vi "Harmonics MSMT Configure 5668 SA Pin.vi"(8 "error in (no error)":errorcluster, 11 "Harmonics in":refnum<class "Harmonics.lvclass">) -> (0 "error out":errorcluster, 2 "Original SA Pin":string, 3 "Harmonics out":refnum<class "Harmonics.lvclass">)   [LabVIEW 2018, in "Harmonics.lvlib" / "Harmonics.lvclass"]
uses:
  Harmonics.lvclass
  C:/Sequence Automation/Plugins/Measurement Interface.lvlibp/Measurement Interface.lvclass
  Plugins/Measurement Interface.lvlibp/Private Methods/Measurement Parameters/Read Measurement Parameters.vi
  Plugins/Measurement Interface.lvlibp/Private Methods/Measurement Parameters/Write Measurement Parameters.vi
  Plugins/String Database.lvlibp/String Database.lvclass
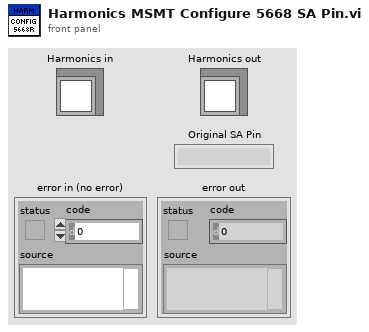
[diagram p1: front panel]
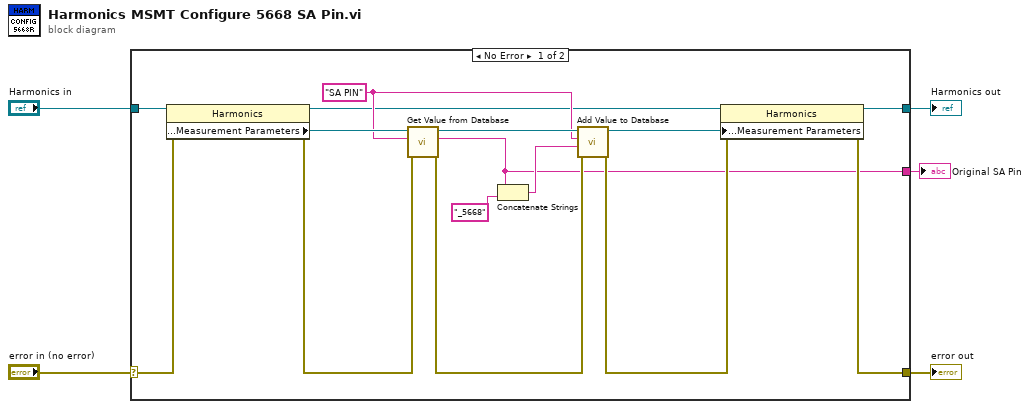
[diagram p0: block diagram]
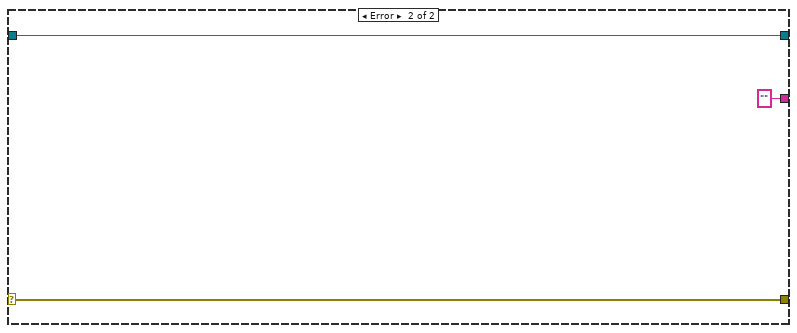
[diagram p2: hidden frame]
diagram:
  n1 = case shown="No Error" "error in (no error)" {
    selector: "error in (no error)" -> [w20 w23]
    tunnel: [w10 w23] -> w4
    tunnel: [w8 w22] -> w2
    tunnel: "Harmonics in" -> [w19 w22]
    tunnel: [w6 "" ("Entry Value")] -> w1
    frame No Error {
      w13 = "SA PIN" ("Entry Name")
      n2 = property class="Harmonics"(reference=w19, error in=w20) -> (reference out=w9:refnum<class "Harmonics.lvclass">, error out=w17:errorcluster, "Protected Methods:Measurement Parameters"=w18:refnum<class "String Database.lvclass">)
      n3 = call "Get Value from Database.vi"("error in (no error)"=w17, "Entry Name"=w13, "Message in"=w18) -> ("error out"=w12:errorcluster, "Entry Value"=w6:string, "Message out"=w15:refnum<class "String Database.lvclass">)  [unwired: 5 in, 1 out]
      n4 = Concatenate Strings(w6, "_5668" ("string")) -> (w14:string)
      n5 = call "Add Value to Database.vi"("error in (no error)"=w12, "Entry Value"=w14, "Entry Name"=w13, "Dictionary In"=w15) -> ("error out"=w11:errorcluster, "Dictionary Out"=w7:refnum<class "String Database.lvclass">)  [unwired: 5 in, 1 out]
      n6 = property class="Harmonics"(reference=w9, error in=w11, "Protected Methods:Measurement Parameters"=w7) -> (reference out=w8:refnum<class "Harmonics.lvclass">, error out=w10:errorcluster)
    }
    frame Error {
    }
  }
  "error out" <- w4
  "Harmonics out" <- w2
  "Original SA Pin" <- w1
